vi "Queuing&ADC_test(1).vi"() -> ()   [LabVIEW 2017]
uses:
  <vilib>/measure/maspectr.llb/Power Spectrum and PSD Export Mode.ctl
  <vilib>/DAQmx/read.llb/DAQmx Read (Analog Wfm 1Chan NSamp).vi
  <vilib>/DAQmx/create/channels.llb/DAQmx Create Channel (AI-Voltage-Basic).vi
  <vilib>/DAQmx/configure/timing.llb/DAQmx Timing (Sample Clock).vi
  <vilib>/DAQmx/miscellaneous.llb/DAQmx Fill In Error Info.vi
  <vilib>/Analysis/3filter.llb/FIR Filter (DBL).vi
  <vilib>/measure/maspectr.llb/FFT Power Spectrum and PSD for 1 Chan.vi
  <vilib>/measure/NI_MAPro.lvlib
  <vilib>/Analysis/NI_AALBase.lvlib
  <vilib>/Analysis/NI_AALPro.lvlib
panel:
  out "RX Signal 5":waveform(dbl)(graph)
  out "RX Signal 4":waveform(dbl)[](graph)
  out "RX Signal 2":waveform(dbl)[](graph)
  in  "Pulse length(sec)":dbl=30000.0 format="%#_6p"
  in  "Frequency2(Hz)":dbl=30000.0 format="%#_6p"
  in  "Frequency1(Hz)":dbl=30000.0 format="%#_6p"
  out "RX Signal":waveform(dbl)(graph)
  out "RX Signal 3":cluster{"f0":dbl, "df":dbl, "magnitude":dbl[]}(graph)
  in  "sample mode":i32(ring)=10123 caption="샘플 모드" items=["유한 샘플"=10178, "연속 샘플"=10123, "하드웨어 타이밍에 의한 단일 포인트"=12522]
  in  "sampling rate":dbl=1000.0 caption="속도" format="%0.2f"
  in  "DAQmx 물리적 채널":tag="PXI2Slot13/ai7"
  in  "DAQmx 디바이스 이름":tag="PXI2Slot13"
  in  "RX Time(sec)":dbl
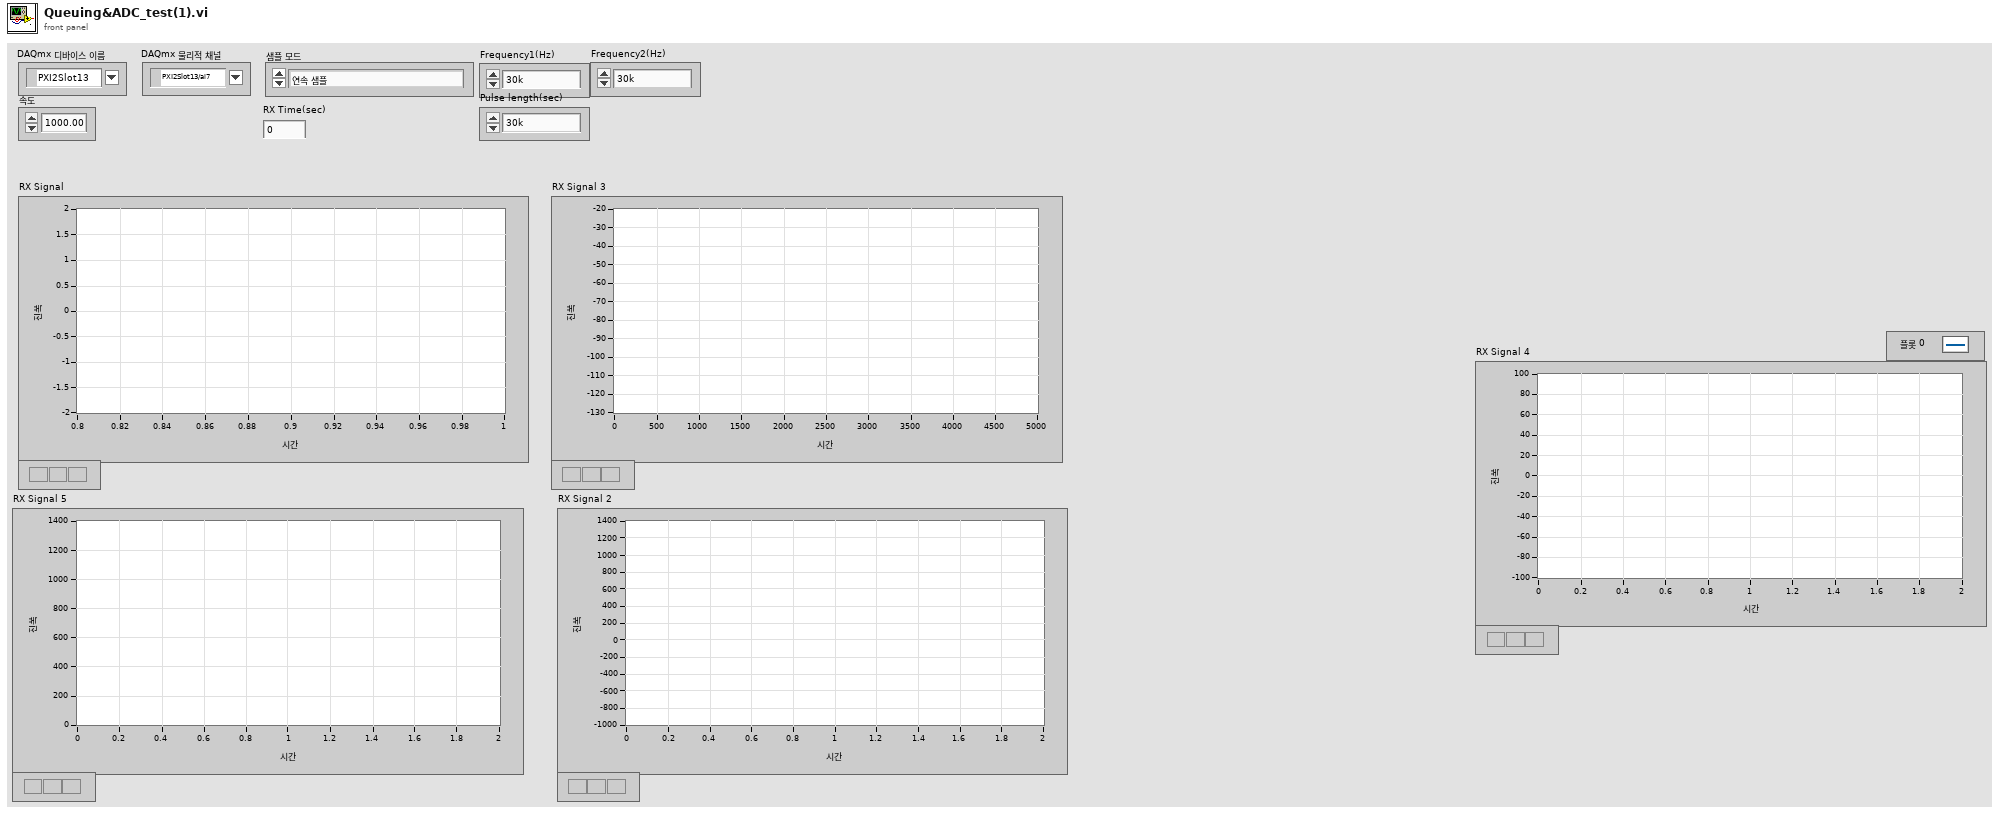
[diagram p1: front panel]
types:
  T1 = typedef "NI_MAPro.lvlib/Power Spectrum and PSD Export Mode.ctl" = u16
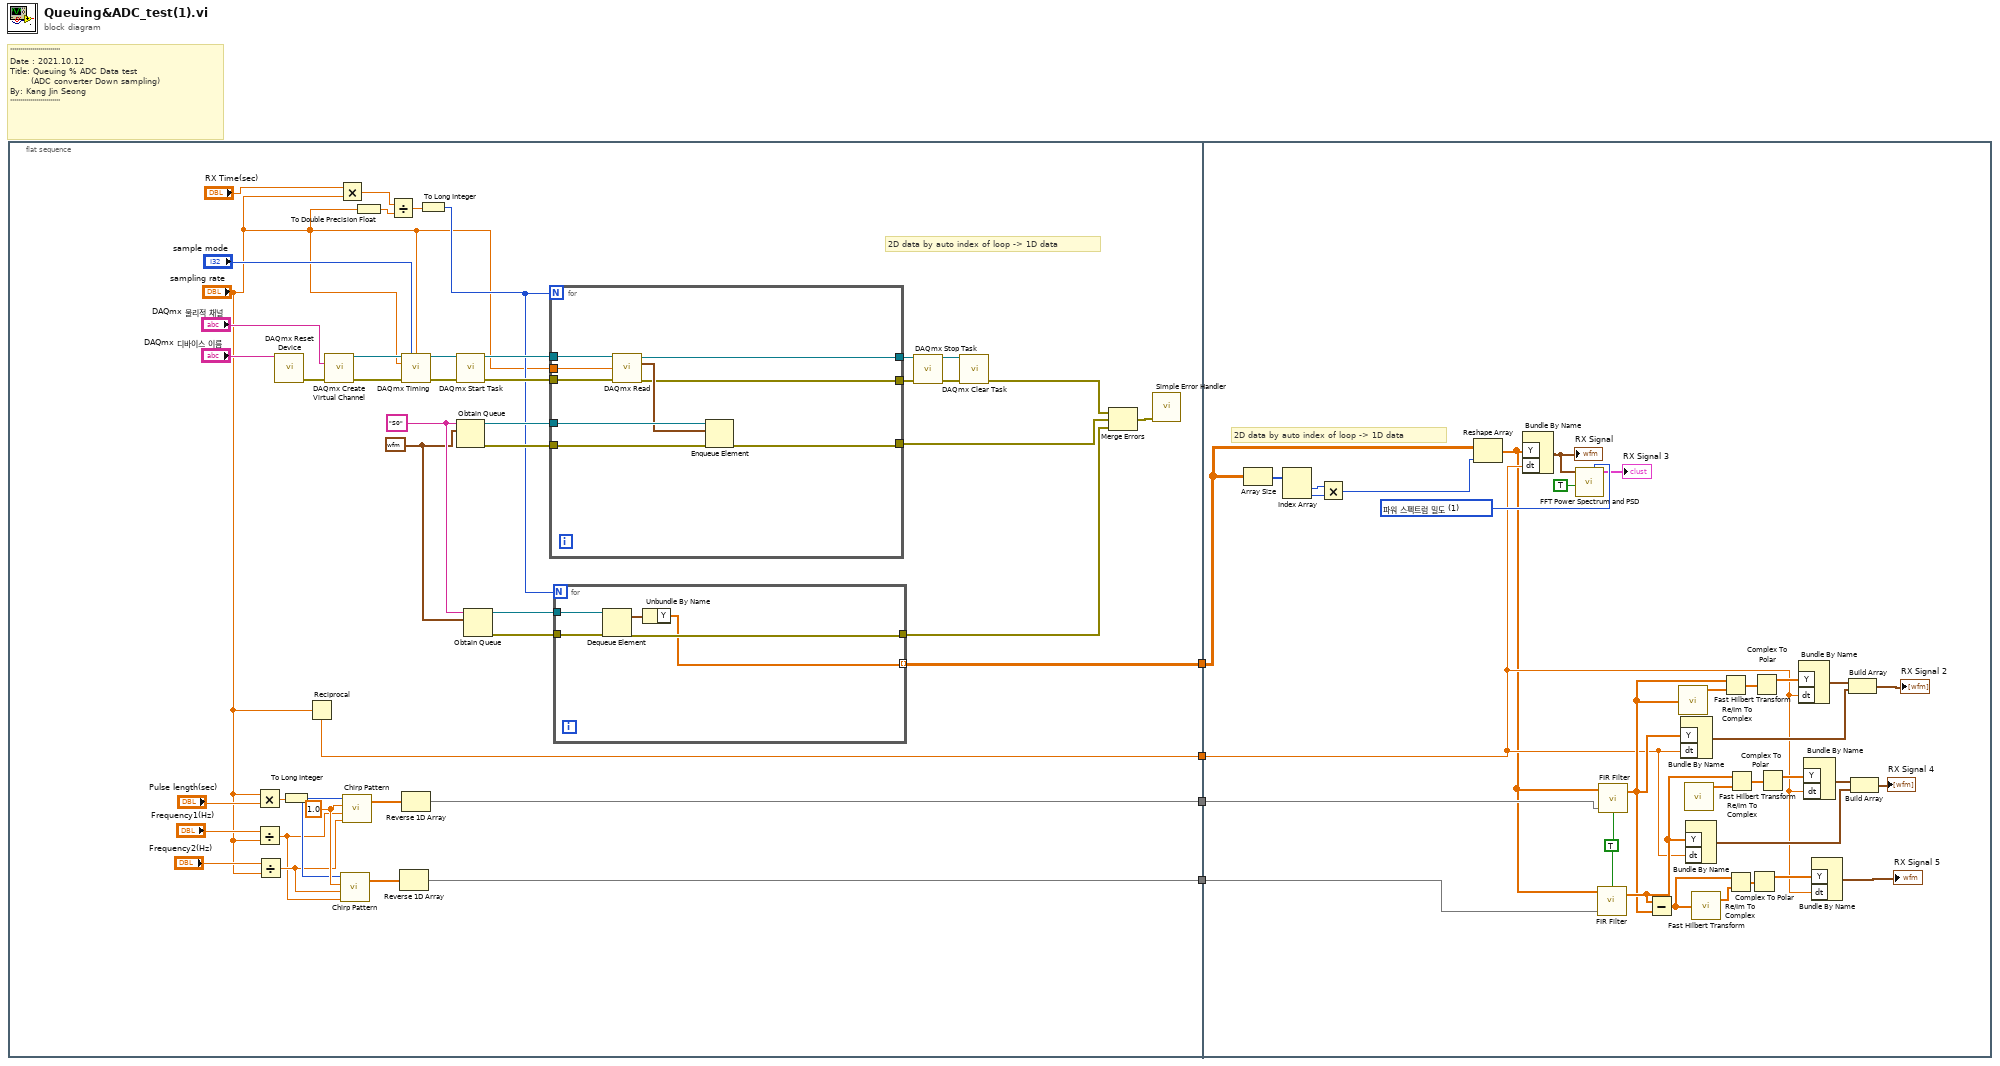
[diagram p0: block diagram]
diagram:
  # "'''''''''''''''''''''''''\nDate : 2021.10.12\nTitle: Queuing % ADC Data test\n       (ADC converter Down sampling)\nBy: Kang Jin Seong\n'''''''''''''''''''''''''"
  n1 = flat-sequence {
    tunnel: [w18] -> w4
    tunnel: [w19] -> w3
    tunnel: [w6] -> w2
    tunnel: [w5] -> w1
    tunnel: w4 -> [w66]
    tunnel: w3 -> [w91]
    tunnel: w2 -> [w65]
    tunnel: w1 -> [w64]
    frame #0 {
      w12 = 1.0 ("amplitude")
      w27 = "S0" ("이름(이름없음)")
      w26 = waveform(dbl) {"t0"=timestamp(0 s since 1904-01-01), "dt"=1.0, "Y"=[]} ("Waveform")
      # "2D data by auto index of loop -> 1D data"
      n2 = Multiply(x="sampling rate", y="Pulse length(sec)") -> (x*y=w16:dbl)
      n3 = Divide(x="Frequency1(Hz)", y="sampling rate") -> (x/y=w9:dbl)
      n4 = Divide(x="Frequency2(Hz)", y="sampling rate") -> (x/y=w10:dbl)
      n5 = call <vilib>:"DAQmx Reset Device.vi"("device in"="DAQmx 디바이스 이름") -> ("error out"=w43:errorcluster)  [unwired: 1 in, 13 out]
      n6 = To Long Integer(number=w16) -> (32bit integer=w11:i32)
      n7 = Reciprocal(x="sampling rate") -> (1/x=w18:dbl)
      n8 = call-poly <vilib>:"DAQmx Create Virtual Channel.vi"("physical channels"="DAQmx 물리적 채널", "error in"=w43) -> ("task out"=w45:refnum<k21>, "error out"=w47:errorcluster)  [unwired: 7 in, 5 out]
      n9 = Multiply(x="RX Time(sec)", y="sampling rate") -> (x*y=w38:dbl)
      n10 = call <vilib>:"Chirp Pattern.vi"("f2"=w9, "f1"=w10, "amplitude"=w12, "samples"=w11) -> ("Chirp Pattern"=w8:dbl[])  [unwired: 1 out]
      n11 = call <vilib>:"Chirp Pattern.vi"("f2"=w10, "f1"=w9, "amplitude"=w12, "samples"=w11) -> ("Chirp Pattern"=w13:dbl[])  [unwired: 1 out]
      n12 = To Double Precision Float(number="sampling rate") -> (double precision float=w37:dbl)
      n13 = Divide(x=w38, y=w37) -> (x/y=w36:dbl)
      n14 = Reverse 1D Array(array=w8) -> (reversed array=w5:dbl[])
      n15 = call-poly <vilib>:"DAQmx Timing.vi"("task/channels in"=w45, "sample mode"="sample mode", "samples per channel"="sampling rate", "rate"="sampling rate", "error in"=w47) -> ("task out"=w48:refnum<k21>, "error out"=w46:errorcluster)  [unwired: 2 in, 7 out]
      n16 = Reverse 1D Array(array=w13) -> (reversed array=w6:dbl[])
      n17 = To Long Integer(number=w36) -> (32bit integer=w20:i32)
      n18 = call <vilib>:"DAQmx Start Task.vi"("task/channels in"=w48, "error in"=w46) -> ("task out"=w31:refnum<k21>, "error out"=w30:errorcluster)  [unwired: 12 in]
      n19 = Obtain Queue(name (unnamed)=w27, element data type=w26) -> (queue out=w35:refnum<queue>, error out=w34:errorcluster)  [unwired: 3 in, 1 out]
      n20 = Obtain Queue(name (unnamed)=w27, element data type=w26) -> (queue out=w25:refnum<queue>, error out=w24:errorcluster)  [unwired: 3 in, 1 out]
      n21 = for {
        N: w20 -> [_]
        tunnel: w35 -> [w62]
        tunnel: w34 -> [w61]
        tunnel: [w60] -> w32
        tunnel: w31 -> [w58]
        tunnel: w30 -> [w57]
        tunnel: [w56] -> w29
        tunnel: [w55] -> w28
        tunnel: "sampling rate" -> [w54]
        n22 = call-poly <vilib>:"DAQmx Read.vi"("task/channels in"=w58, "number of samples per channel"=w54, "error in"=w57) -> ("task out"=w56:refnum<k21>, "data"=w59:waveform(dbl), "error out"=w55:errorcluster)  [unwired: 10 out]
        n23 = Enqueue Element(queue=w62, element=w59, error in (no error)=w61) -> (error out=w60:errorcluster)  [unwired: 1 in, 2 out]
      }
      n24 = for {
        N: w20 -> [_]
        tunnel: w25 -> [w53]
        tunnel: w24 -> [w52]
        tunnel: [w51] -> w23
        tunnel: [w49] -> w19 mode=indexing
        n25 = Dequeue Element(queue=w53, error in (no error)=w52) -> (element=w50:waveform(dbl), error out=w51:errorcluster)  [unwired: 1 in, 2 out]
        n26 = Unbundle By Name(w50) -> ("Y"=w49:dbl[])
      }
      n27 = call <vilib>:"DAQmx Stop Task.vi"("task/channels in"=w29, "error in"=w28) -> ("task out"=w41:refnum<k21>, "error out"=w42:errorcluster)  [unwired: 12 out]
      n28 = call <vilib>:"DAQmx Clear Task.vi"("task in"=w41, "error in"=w42) -> ("error out"=w33:errorcluster)  [unwired: 13 out]
      n29 = Merge Errors(w33, w32, w23) -> (w22:errorcluster)
      n30 = call <vilib>:"Simple Error Handler.vi"("error in (no error)"=w22) -> ()  [unwired: 4 in, 5 out]
    }
    frame #1 {
      w67 = TRUE ("init/cont (init:F)")
      w89 = T1 1 items=["파워 스펙트럼", "파워 스펙트럼 밀도"] ("export mode")
      # "2D data by auto index of loop -> 1D data"
      n31 = Array Size(array=w91) -> (size(s)=w92:i32[])
      n32 = Index Array(array=w92) -> (element #1=w94:i32, element #2=w93:i32)  [unwired: 2 in]
      n33 = Multiply(x=w94, y=w93) -> (x*y=w95:i32)
      n34 = Reshape Array(w91, w95) -> (w63:dbl[])
      n35 = Bundle By Name("Y"=w63, "dt"=w66) -> (w90:waveform(dbl))  [unwired: 1 in]
      "RX Signal" <- w90
      n36 = call-poly <vilib>:"FFT Power Spectrum and PSD.vi"("export mode"=w89, "dB On (F)"=TRUE, "time signal"=w90) -> ("Power Spectrum / PSD"=→"RX Signal 3":cluster{"f0":dbl, "df":dbl, "magnitude":dbl[]})  [unwired: 5 in, 3 out]
      n37 = call-poly <vilib>:"FIR Filter.vi"("init/cont (init:F)"=w67, "FIR Coefficients"=w64, "X"=w63) -> ("Filtered X"=w71:dbl[])  [unwired: 1 in, 1 out]
      n38 = call-poly <vilib>:"FIR Filter.vi"("init/cont (init:F)"=w67, "FIR Coefficients"=w65, "X"=w63) -> ("Filtered X"=w70:dbl[])  [unwired: 1 in, 1 out]
      n39 = Subtract(x=w71, y=w70) -> (x-y=w69:dbl[])
      n40 = call <vilib>:"Fast Hilbert Transform.vi"("X"=w70) -> ("Hilbert{X}"=w86:dbl[])  [unwired: 1 out]
      n41 = Bundle By Name("Y"=w70, "dt"=w66) -> (w82:waveform(dbl))  [unwired: 1 in]
      n42 = call <vilib>:"Fast Hilbert Transform.vi"() -> ("Hilbert{X}"=w80:dbl[])  [unwired: 1 in, 1 out]
      n43 = Bundle By Name("Y"=w71, "dt"=w66) -> (w76:waveform(dbl))  [unwired: 1 in]
      n44 = call <vilib>:"Fast Hilbert Transform.vi"("X"=w69) -> ("Hilbert{X}"=w74:dbl[])  [unwired: 1 out]
      n45 = Re/Im To Complex(1:w86, 2:w70) -> (0:w85:cdb[])
      n46 = Re/Im To Complex(1:w74, 2:w69) -> (0:w73:cdb[])
      n47 = Re/Im To Complex(1:w80, 2:w71) -> (0:w79:cdb[])
      n48 = Complex To Polar(r * e^(i*theta)=w73) -> (r=w72:dbl[])  [unwired: 1 out]
      n49 = Complex To Polar(r * e^(i*theta)=w85) -> (r=w84:dbl[])  [unwired: 1 out]
      n50 = Complex To Polar(r * e^(i*theta)=w79) -> (r=w78:dbl[])  [unwired: 1 out]
      n51 = Bundle By Name("Y"=w84, "dt"=w66) -> (w83:waveform(dbl))  [unwired: 1 in]
      n52 = Bundle By Name("Y"=w78, "dt"=w66) -> (w77:waveform(dbl))  [unwired: 1 in]
      n53 = Bundle By Name("Y"=w72, "dt"=w66) -> (→"RX Signal 5":waveform(dbl))  [unwired: 1 in]
      n54 = Build Array(w83, w82) -> (→"RX Signal 2":waveform(dbl)[])
      n55 = Build Array(w77, w76) -> (→"RX Signal 4":waveform(dbl)[])
    }
  }
